vi "NIRFSG_Open.vi"(0 "Session Name":refnum<k15>, 5 "Reset Instr":bool, 7 "Open Session":bool, 11 "error in (no error)":errorcluster) -> (4 "instrument handle out":refnum<k15>, 15 "error out":errorcluster)   [LabVIEW 2015]
uses:
  <instrlib>/niRFSG/niRFSG.llb/niRFSG Ref Clock Sources.ctl
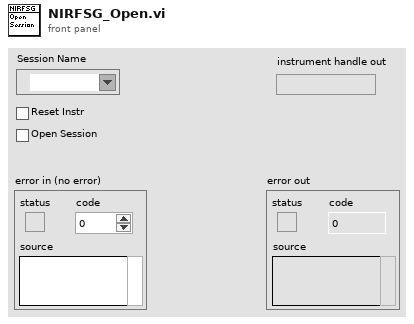
[diagram p1: front panel]
types:
  T1 = typedef "niRFSG Ref Clock Sources.ctl" = string
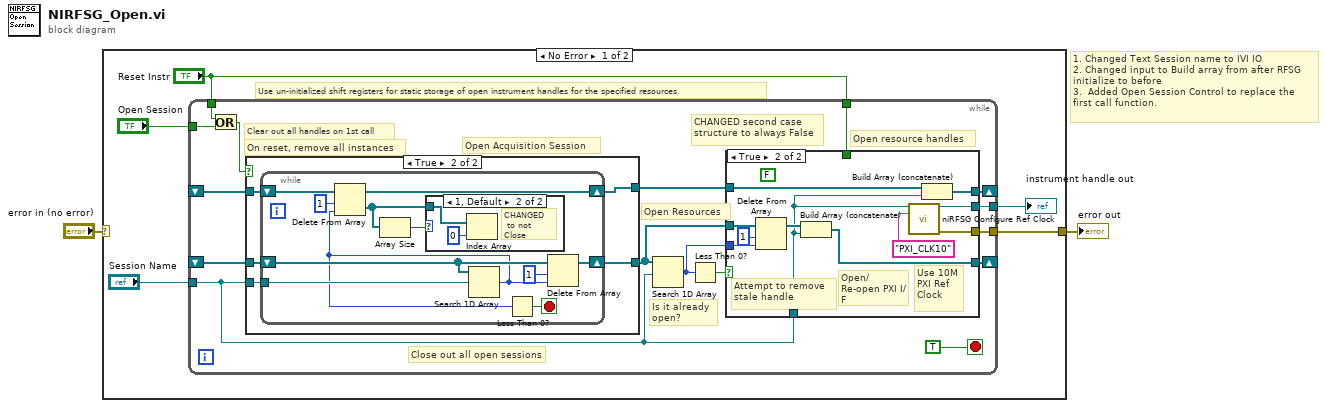
[diagram p0: block diagram]
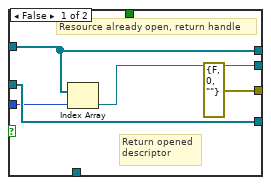
[diagram p4: hidden frame]
diagram:
  # "1. Changed Text Session name to IVI IO\n2. Changed input to Build array from after RFSG initialize to before\n3.  Added Open Session Control to replace the first call function."
  n1 = case shown="No Error" "error in (no error)" {
    selector: "error in (no error)" -> [_ w60]
    tunnel: [w6 w60] -> w1
    frame No Error {
      # "Use un-initialized shift registers for static storage of open instrument handles for the specified resources."
      n2 = while {
        shift-right: [w23] -> _
        shift-left: _ -> [w10]
        shift-right: [w22] -> _
        shift-left: _ -> [w11]
        tunnel: "Session Name" -> [w16]
        tunnel: [w20] -> w6
        tunnel: "Reset Instr" -> [w19]
        tunnel: [w18] -> w7
        tunnel: "Reset Instr" -> [w12]
        tunnel: "Open Session" -> [w9]
        stop <- TRUE stop-if-true
        # "CHANGED second case\nstructure to always False"
        # "Close out all open sessions"
        # "Open resource handles"
        # "On reset, remove all instances"
        # "Clear out all handles on 1st call"
        # "Open Acquisition Session"
        # "Is it already open?"
        # "Open Resources"
        n3 = Or(x=w12, y=w9) -> (x .or. y?=w13:bool)
        n4 = case shown="True" w13 {
          tunnel: w10 -> [w24 w29]
          tunnel: w11 -> [w25 w30]
          tunnel: w16 -> [_ w28]
          tunnel: [w24 w27] -> w15
          tunnel: [w25 w26] -> w14
          frame False {
            # "No Reset"
          }
          frame True {
            n5 = while {
              shift-right: [w36] -> w26
              shift-left: w30 -> [w35]
              shift-right: [w38] -> w27
              shift-left: w29 -> [w32]
              tunnel: w28 -> [w41]
              stop <- w40 stop-if-true
              n6 = Search 1D Array(1D array=w32, element=w41) -> (index of element=w31:i32)  [unwired: 1 in]
              n7 = Delete From Array(array=w35, length=1, index=w31) -> (deleted portion=w33:refnum<k15>[], array with subset deleted=w36:refnum<k15>[])
              n8 = Array Size(array=w33) -> (size(s)=w34:i32)
              n9 = case shown="1, Default" w34 {
                tunnel: w33 -> [_ w42]
                frame 0 {
                }
                frame 1, Default {
                  # "CHANGED \n to not Close"
                  n10 = Index Array(array=w42, index=0) -> ()  [unwired: 1 out]
                }
              }
              n11 = Less Than 0?(x=w31) -> (x < 0?=w40:bool)
              n12 = Delete From Array(array=w32, length=1, index=w31) -> (array with subset deleted=w38:refnum<k15>[])  [unwired: 1 out]
            }
          }
        }
        n13 = Search 1D Array(1D array=w15, element=w16) -> (index of element=w21:i32)  [unwired: 1 in]
        n14 = Less Than 0?(x=w21) -> (x < 0?=w8:bool)
        n15 = case shown="True" w8 {
          tunnel: w15 -> [w48 w58]
          tunnel: w16 -> [_ w49]
          tunnel: [w48 w59] -> w23
          tunnel: [w45 w54] -> w22
          tunnel: w21 -> [w47 w56]
          tunnel: w14 -> [w45 w53]
          tunnel: [errorcluster {"status"=FALSE, "code"=0, "source"=""} ("error out") w52] -> w20
          tunnel: w19 -> [_ _]
          tunnel: [w46 w51] -> w18
          frame False {
            # "Resource already open, return handle"
            # "Return opened\ndescriptor"
            n16 = Index Array(array=w45, index=w47) -> (element=w46:refnum<k15>)
          }
          frame True {
            (unwired) FALSE ("ID Query")
            # "Use 10M\nPXI Ref\nClock"
            # "Attempt to remove\nstale handle"
            # "Open/Re-open PXI I/F"
            n17 = Delete From Array(array=w58, length=1, index=w56) -> (array with subset deleted=w57:refnum<k15>[])  [unwired: 1 out]
            n18 = Build Array (concatenate)(w57, w49) -> (w59:refnum<k15>[])
            n19 = call <instrlib>:"niRFSG Configure Ref Clock.vi"("instrument handle"=w49, "ref clock source"=T1 "PXI_CLK10" ("clock source")) -> ("instrument handle out"=w51:refnum<k15>, "error out"=w52:errorcluster)  [unwired: 12 in]
            n20 = Build Array (concatenate)(w53, w49) -> (w54:refnum<k15>[])
          }
        }
      }
      "instrument handle out" <- w7
    }
    frame Error {
    }
  }
  "error out" <- w1
